vi "GlobalVars.vi"() -> ()   [LabVIEW 2016]
panel:
  out "STATE":bool
  # "0 - WAITING TO READ BALL"
  # "1 - WAITING TO READ PATTERN"
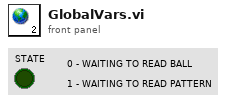
[diagram p1: front panel]
diagram:
